vi "main.vi"() -> ()   [LabVIEW 2011]
panel:
  out "String":string
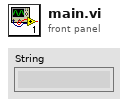
[diagram p1: front panel]
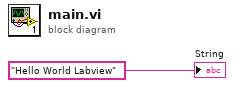
[diagram p0: block diagram]
diagram:
  "String" <- "Hello World Labview"
